vi "Motors On.vi"(8 "error in (no error)":errorcluster, 11 ".NET Refnum in":refnum<k24>) -> (0 "error out":errorcluster, 3 ".NET Refnum out":refnum<k24>)   [LabVIEW 2019, in "ESP301.lvlib"]
uses:
  ESP301.lvlib
  Newport.ESP301.CommandInterface
  <vilib>/Utility/config.llb/Read Key (I32).vi
  <vilib>/Utility/config.llb/NI_LVConfig.lvlib
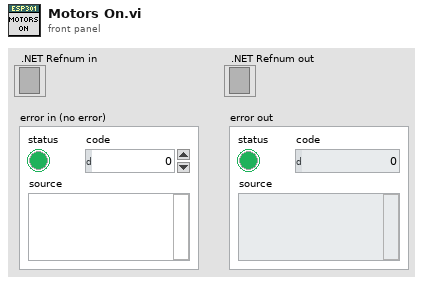
[diagram p1: front panel]
types:
  T1 = typedef "NI_LVConfig.lvlib/Config Data RefNum.ctl" = refnum<k1>
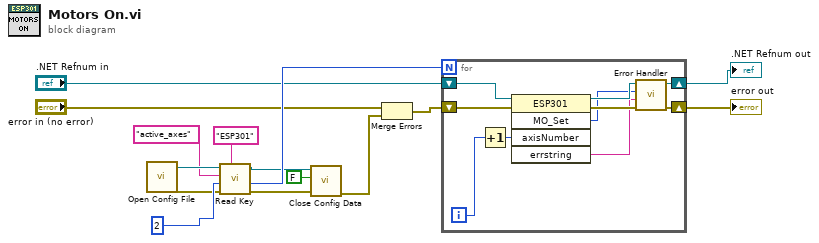
[diagram p0: block diagram]
diagram:
  n1 = call "Open Config File.vi"() -> ("error out"=w7:errorcluster, "Refnum out"=w8:T1)  [unwired: 10 in]
  n2 = call-poly <vilib>:"Read Key.vi"("section"="ESP301", "error in (no error)"=w7, "default value"=2, "key"="active_axes", "refnum"=w8) -> ("error out"=w11:errorcluster, "value"=w15:i32, "refnum out"=w10:T1)  [unwired: 3 in, 1 out]
  n3 = call <vilib>:"Close Config Data.vi"("error in (no error)"=w11, "write file if changed (T)"=FALSE, "refnum"=w10) -> ("error out"=w13:errorcluster)  [unwired: 7 in, 1 out]
  n4 = Merge Errors("error in (no error)", w13) -> (w12:errorcluster)
  n5 = for {
    N: w15 -> [_]
    shift-right: [w22] -> w4
    shift-left: ".NET Refnum in" -> [w25]
    shift-right: [w23] -> w3
    shift-left: w12 -> [w18]
    i -> [w17]
    n6 = Increment(x=w17) -> (x+1=w16:i32)
    n7 = invoke class="ESP301" method="MO_Set"(reference=w25, error in=w18, "axisNumber"=w16) -> (reference out=w21:refnum<k24>, error out=w24:errorcluster, "MO_Set"=w19:i32, "errstring"=w20:string)  [unwired: 2 in, 1 out]
    n8 = call "Error Handler.vi"("error in (no error)"=w24, "value"=w20, "OpenInstrument"=w19, ".NET Refnum in"=w21) -> ("error out"=w23:errorcluster, ".NET Refnum out"=w22:refnum<k24>)  [unwired: 6 in]
  }
  ".NET Refnum out" <- w4
  "error out" <- w3
